vi "getSession.vi"(11 "Client in":refnum<class "Client.lvclass">) -> (1 "valid?":bool, 2 "Session":refnum<class "Session.Client.lvclass">, 3 "Client out":refnum<class "Client.lvclass">)   [LabVIEW 2013, in "MQTT Client.lvlib" / "Client.lvclass"]
uses:
  Client.lvclass
  Session.Client/Session.Client.lvclass
  Client.lvclass/Client.ctl
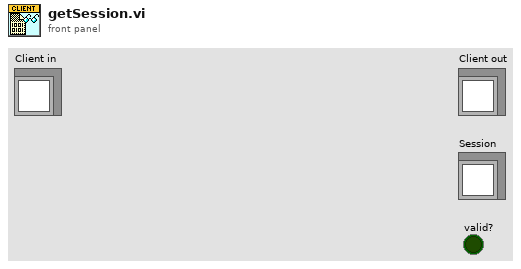
[diagram p1: front panel]
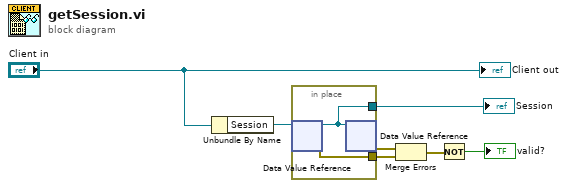
[diagram p0: block diagram]
diagram:
  n1 = Unbundle By Name("Client in") -> ("Session"=w6:refnum<data-value>)
  n2 = in-place {
    in-place-border: [w9] -> w4
    in-place-border: [w8] -> w2
    n3 = in-place-dvr #1(w6) -> (w8:refnum<class "Session.Client.lvclass">, w9:errorcluster)
    n4 = in-place-dvr #1(w8) -> (w5:errorcluster)  [unwired: 1 out]
  }
  "Session" <- w2
  n5 = Merge Errors(w5, w4) -> (w3:errorcluster)
  n6 = Not(x=w3) -> (.not. x?=→"valid?":bool)
  "Client out" <- "Client in"
